vi "Write Pixel (H).vi"(8 "error in (no error)":errorcluster, 10 "Pixel (H)":u32, 11 "Camera in":refnum<class "Camera.lvclass">) -> (0 "error out":errorcluster, 3 "Camera out":refnum<class "Camera.lvclass">)   [LabVIEW 2018, in "Camera.lvlib" / "Camera.lvclass"]
uses:
  Camera.lvclass
  Camera.lvclass/Camera.ctl
  Custom Controls/Camera Setting.ctl
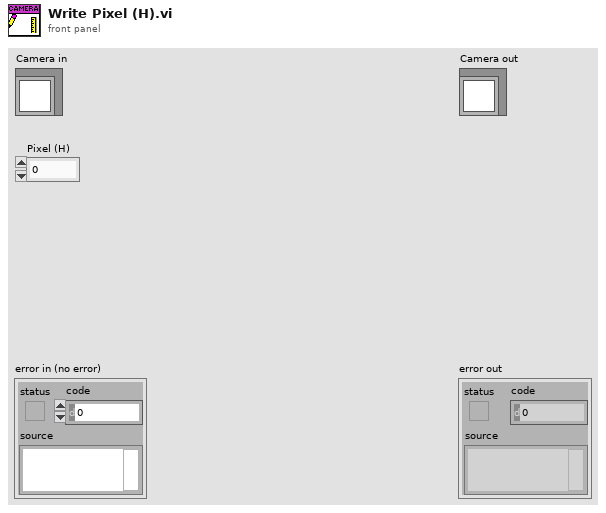
[diagram p1: front panel]
types:
  T1 = typedef "Camera.lvlib/Camera.lvclass/Camera Setting.ctl" = enum16{"Brightness", "Rotation", "Contrast", "Exposure", "Frame Rate", "Gain", "Gamma", "Pixel(H)", "Pixel(W)", "Sharpness"}
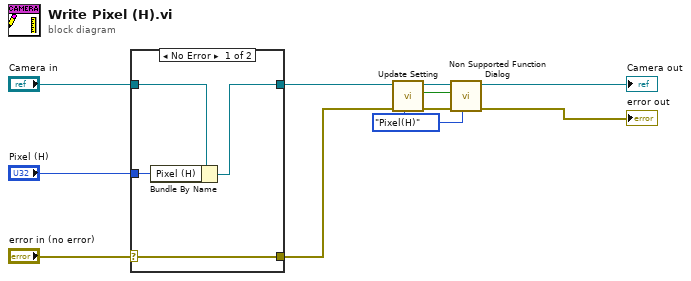
[diagram p0: block diagram]
diagram:
  w2 = Camera_Setting."Pixel(H)" ("Update Setting:")
  n1 = case shown="No Error" "error in (no error)" {
    selector: "error in (no error)" -> [w15 w16]
    tunnel: [w15 w16] -> w6
    tunnel: [w13 w17] -> w8
    tunnel: "Camera in" -> [w14 w17]
    tunnel: "Pixel (H)" -> [w12 _]
    frame No Error {
      n2 = Bundle By Name(cluster=w14, "Pixel (H)"=w12) -> (w13:refnum<class "Camera.lvclass">)
    }
    frame Error {
    }
  }
  n3 = call-dynamic "Update Setting.vi"("Update Setting:"=w2, "error in"=w6, "Camera in"=w8) -> ("error out"=w4:errorcluster, "Supported?"=w1:bool, "Camera out"=w7:refnum<class "Camera.lvclass">)  [unwired: 6 in]
  n4 = call "Non Supported Function Dialog.vi"("Update Setting:"=w2, "error in"=w4, "Supported?"=w1, "Camera in"=w7) -> ("error out"=→"error out":errorcluster, "Camera out"=→"Camera out":refnum<class "Camera.lvclass">)  [unwired: 6 in]
